vi "FTW-JSON-Format-Timestamp.vi"(1 "LabVIEW Timestamp":timestamp format="%^<%Y-%m-%dT%H:%M:%S%3uZ>T") -> (0 "JSON String":string)   [LabVIEW 2015]
uses:
  Time/FTW-Time-DisplayFormat-Timestamp.ctl
panel:
  # "Inputs"
  # "Outputs"
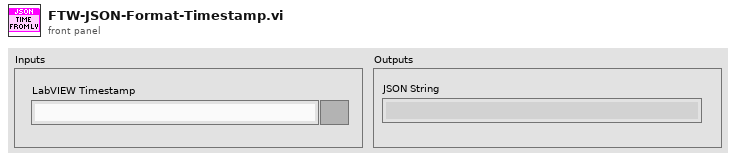
[diagram p1: front panel]
types:
  T1 = typedef "FTW-Time-DisplayFormat-Timestamp.ctl" = enum16{"YYYY-MM-DDT00:00:00.000Z (UTC)", "YYYY-MM-DDT00:00:00.000 (locale)", "YYYY-MM-DDT00:00:00.000+hh:mm (time zone)", "YYYY-MM-DDT00-00-00Z (simple UTC)", "YYYY-MM-DDT00-00-00 (simple locale)", "YYYY-MM-DD"}
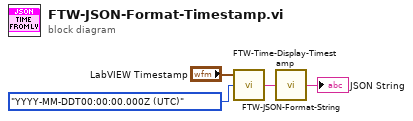
[diagram p0: block diagram]
diagram:
  n1 = call "FTW-Time-Display-Timestamp.vi"("Format"=FTW-Time-DisplayFormat-Timestamp."YYYY-MM-DDT00:00:00.000Z (UTC)", "Timestamp (unwired for current time)"="LabVIEW Timestamp") -> ("Formatted Timestamp"=w3:string)  [unwired: 2 in]
  n2 = call "FTW-JSON-Format-String.vi"("LabVIEW String"=w3) -> ("JSON String"=→"JSON String":string)
